vi "Dingle fitter.vi"(0 "1/B":dbl[](array[numeric]) format="%.2f", 1 "experiment":u16(ring) items=["2D SdH", "2D dHvA (dM/dt)", "2D dHvA (dM/dB)", "2D dHvA (M)", "2D dHvA (torque)", "3D SdH", "3D dHvA (dM/dt)", "3D dHvA (dM/dB)", "3D dHvA (M)", "3D dHvA (torque)"], 2 "amp.":dbl[](array[numeric]) format="%.2f", 3 "dB/dt":dbl[](array[numeric]) format="%.2f", 4 "T":dbl format="%.3f", 8 "m*":dbl[](array[numeric]) format="%.2f") -> (5 "gamma":dbl format="%.2f", 6 "ln [A]":dbl format="%.2f", 7 "sum of square deviations":dbl format="%.2f")   [LabVIEW 2016]
uses:
  <vilib>/Analysis/NI_AALPro.lvlib
panel:
  out "plotted data":cluster{dbl[], dbl[]}[](graph)
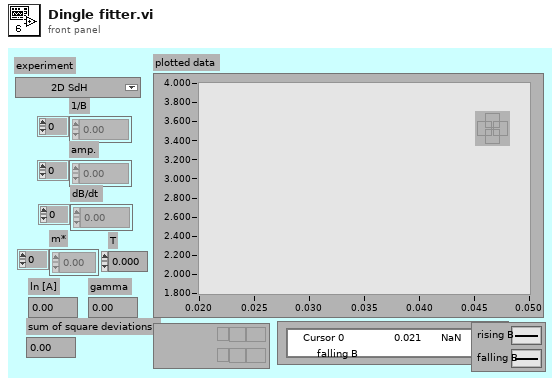
[diagram p1: front panel]
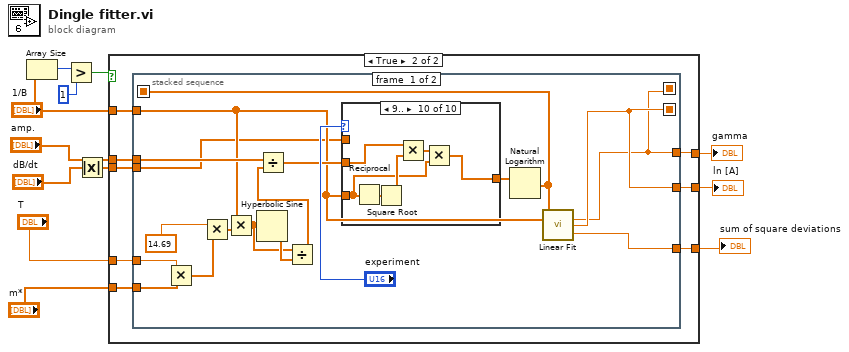
[diagram p0: block diagram]
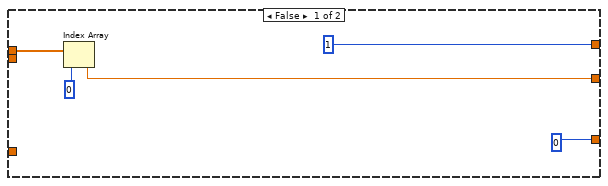
[diagram p2: hidden frame]
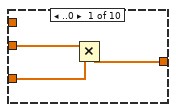
[diagram p3: hidden frame]
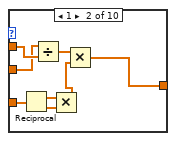
[diagram p4: hidden frame]
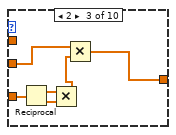
[diagram p5: hidden frame]
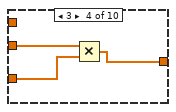
[diagram p6: hidden frame]
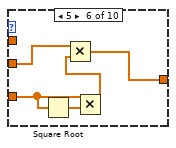
[diagram p8: hidden frame]
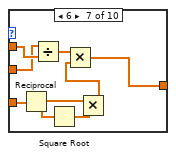
[diagram p9: hidden frame]
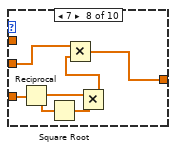
[diagram p10: hidden frame]
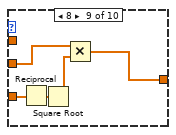
[diagram p11: hidden frame]
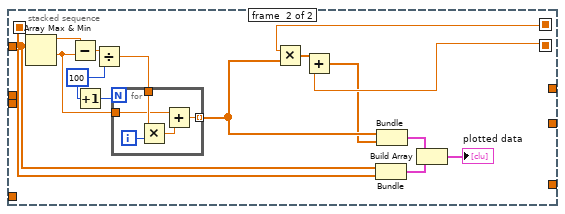
[diagram p12: hidden frame]
diagram:
  n1 = Array Size(array="1/B") -> (size(s)=w10:i32)
  n2 = Greater?(x=w10, y=1) -> (0:w9:bool)
  n3 = Absolute Value(x="dB/dt") -> (abs(x)=w1:dbl[])
  n4 = case shown="True" w9 {
    tunnel: [1 w22] -> w8
    tunnel: "1/B" -> [_ w25]
    tunnel: "amp." -> [w15 w24]
    tunnel: "T" -> [_ w23]
    tunnel: [w14 w21] -> w5
    tunnel: [0 w20] -> w4
    tunnel: w1 -> [_ w19]
    tunnel: "m*" -> [_ w18]
    frame False {
      n5 = Index Array(array=w15, index=0) -> (element=w14:dbl)
    }
    frame True {
      n6 = stacked-sequence {
        seq-local: [w39 _] -> [_ w102]
        seq-local: [w42 _] -> [_ w96]
        seq-local: [w40 _] -> [_ w93]
        tunnel: w25 -> [w35 w94]
        tunnel: w24 -> [w38 _]
        tunnel: w23 -> [w30 _]
        tunnel: [w39 _] -> w22
        tunnel: [w42 _] -> w21
        tunnel: [w41 _] -> w20
        tunnel: w19 -> [w33 _]
        tunnel: w18 -> [w32 _]
        frame #0 {
          n7 = Multiply(x=w30, y=w32) -> (x*y=w31:dbl[])
          n8 = Multiply(x=14.69, y=w31) -> (x*y=w43:dbl[])
          n9 = Multiply(x=w35, y=w43) -> (x*y=w27:dbl[])
          n10 = Hyperbolic Sine(1:w27) -> (0:w28:dbl[])
          n11 = Divide(x=w27, y=w28) -> (x/y=w26:dbl[])
          n12 = Divide(x=w38, y=w26) -> (x/y=w36:dbl[])
          n13 = case shown="9.." "experiment" {
            tunnel: w36 -> [w46 w51 w57 w61 w62 w66 w73 w76 w84 w92]
            tunnel: w35 -> [w44 w53 w58 w60 _ w64 w75 w81 w86 w88]
            tunnel: [w45 w47 w54 w59 w62 w67 w71 w80 w85 w87] -> w34
            tunnel: w33 -> [_ w52 _ _ _ _ w74 _ _ _]
            frame ..0 {
              n14 = Multiply(x=w46, y=w44) -> (x*y=w45:dbl[])
            }
            frame 1 {
              n15 = Reciprocal(x=w53) -> (1/x=w49:dbl[])
              n16 = Divide(x=w51, y=w52) -> (x/y=w50:dbl[])
              n17 = Multiply(x=w49, y=w49) -> (x*y=w48:dbl[])
              n18 = Multiply(x=w50, y=w48) -> (x*y=w47:dbl[])
            }
            frame 2 {
              n19 = Reciprocal(x=w58) -> (1/x=w56:dbl[])
              n20 = Multiply(x=w56, y=w56) -> (x*y=w55:dbl[])
              n21 = Multiply(x=w57, y=w55) -> (x*y=w54:dbl[])
            }
            frame 3 {
              n22 = Multiply(x=w61, y=w60) -> (x*y=w59:dbl[])
            }
            frame 4 {
            }
            frame 5 {
              n23 = Square Root(x=w64) -> (sqrt(x)=w65:dbl[])
              n24 = Multiply(x=w64, y=w65) -> (x*y=w63:dbl[])
              n25 = Multiply(x=w66, y=w63) -> (x*y=w67:dbl[])
            }
            frame 6 {
              n26 = Reciprocal(x=w75) -> (1/x=w69:dbl[])
              n27 = Divide(x=w73, y=w74) -> (x/y=w72:dbl[])
              n28 = Square Root(x=w69) -> (sqrt(x)=w70:dbl[])
              n29 = Multiply(x=w69, y=w70) -> (x*y=w68:dbl[])
              n30 = Multiply(x=w72, y=w68) -> (x*y=w71:dbl[])
            }
            frame 7 {
              n31 = Reciprocal(x=w81) -> (1/x=w78:dbl[])
              n32 = Square Root(x=w78) -> (sqrt(x)=w79:dbl[])
              n33 = Multiply(x=w78, y=w79) -> (x*y=w77:dbl[])
              n34 = Multiply(x=w76, y=w77) -> (x*y=w80:dbl[])
            }
            frame 8 {
              n35 = Reciprocal(x=w86) -> (1/x=w83:dbl[])
              n36 = Square Root(x=w83) -> (sqrt(x)=w82:dbl[])
              n37 = Multiply(x=w84, y=w82) -> (x*y=w85:dbl[])
            }
            frame 9.. {
              n38 = Reciprocal(x=w88) -> (1/x=w91:dbl[])
              n39 = Square Root(x=w91) -> (sqrt(x)=w90:dbl[])
              n40 = Multiply(x=w92, y=w90) -> (x*y=w89:dbl[])
              n41 = Multiply(x=w89, y=w88) -> (x*y=w87:dbl[])
            }
          }
          n42 = Natural Logarithm(1:w34) -> (0:w40:dbl[])
          n43 = call <vilib>:"Linear Fit.vi"("Y"=w40, "X"=w35) -> ("slope"=w39:dbl, "intercept"=w42:dbl, "residue"=w41:dbl)  [unwired: 9 in, 2 out]
        }
        frame #1 {
          w106 = 100
          n44 = Array Max & Min(array=w94) -> (max value=w108:dbl, min value=w103:dbl)  [unwired: 2 out]
          n45 = Subtract(x=w108, y=w103) -> (x-y=w107:dbl)
          n46 = Increment(x=w106) -> (x+1=w105:i32)
          n47 = Divide(x=w107, y=w106) -> (x/y=w104:dbl)
          n48 = for {
            N: w105 -> [_]
            tunnel: w104 -> [w113]
            tunnel: w103 -> [w110]
            tunnel: [w109] -> w98 mode=indexing
            i -> [w112]
            n49 = Multiply(x=w113, y=w112) -> (x*y=w111:dbl)
            n50 = Add(x=w110, y=w111) -> (x+y=w109:dbl)
          }
          n51 = Multiply(x=w102, y=w98) -> (x*y=w97:dbl[])
          n52 = Add(x=w97, y=w96) -> (x+y=w95:dbl[])
          n53 = Bundle("1/B"=w94, w93) -> (w100:cluster{"1/B":dbl[], dbl[]})  [unwired: 1 in]
          n54 = Bundle(w98, w95) -> (w101:cluster{dbl[], dbl[]})  [unwired: 1 in]
          n55 = Build Array(w101, w100) -> (→"plotted data":cluster{"1/B":dbl[], dbl[]}[])
        }
      }
    }
  }
  "gamma" <- w8
  "ln [A]" <- w5
  "sum of square deviations" <- w4
